vi "DetectTransition(LowToHigh).vi"(7 "First Call?: T/F":bool, 11 "InputSignal":bool) -> (3 "RaisingFrontDetected":bool)   [LabVIEW 2013]
doc: "Generate a pulse at the output when the input signal commutate from low to high"
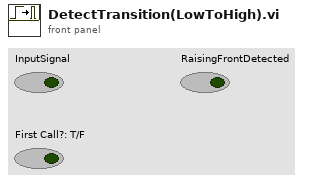
[diagram p1: front panel]
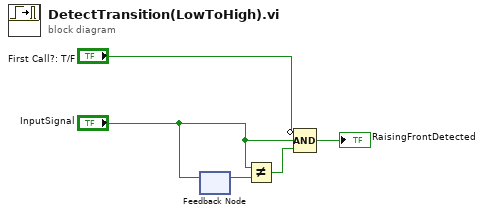
[diagram p0: block diagram]
diagram:
  n1 = feedback #1() -> (w5:bool)  [unwired: 1 in]
  n2 = feedback-in #1("InputSignal") -> ()
  n3 = Not Equal?(x="InputSignal", y=w5) -> (x != y?=w2:bool)
  n4 = Compound Arithmetic op=AND(invert "First Call?: T/F", "InputSignal", w2) -> (→"RaisingFrontDetected":bool)
